vi "17.vi"() -> ()   [LabVIEW 2021]
panel:
  out "Length":i32
  in  "Numeric":i32
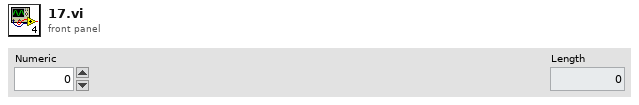
[diagram p1: front panel]
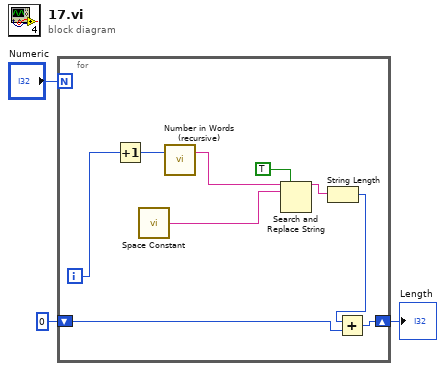
[diagram p0: block diagram]
diagram:
  n1 = for {
    N: "Numeric" -> [_]
    shift-right: [w6] -> w1
    shift-left: 0 -> [w4]
    i -> [w12]
    n2 = Increment(x=w12) -> (x+1=w11:i32)
    n3 = call <vilib>:"Space Constant.vi"() -> ("String"=w9:string)
    n4 = call "Number in Words (recursive).vi"("Number"=w11) -> ("Number in Words"=w10:string)  [unwired: 2 in]
    n5 = Search and Replace String(replace all?=TRUE ("replace all? (F)"), input string=w10, search string=w9) -> (result string=w8:string)  [unwired: 5 in, 3 out]
    n6 = String Length(string=w8) -> (length=w5:i32)
    n7 = Add(x=w5, y=w4) -> (x+y=w6:i32)
  }
  "Length" <- w1
